vi "ex7-15.vi"() -> ()   [LabVIEW 2013]
panel:
  out "subarray":dbl[](array[numeric])
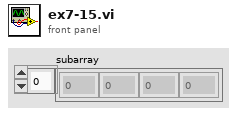
[diagram p1: front panel]
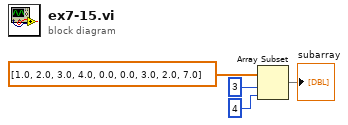
[diagram p0: block diagram]
diagram:
  n1 = Array Subset(array=dbl[] [1.0, 2.0, 3.0, 4.0, 0.0, 0.0, 3.0, 2.0, 7.0], index=3, length=4) -> (→"subarray":dbl[])
